vi "Create Framework Configuration.vi"(11 "Plugins":T5(array[cluster])=[{"plugin components"=[], "group configs"=[], "plugin timing"={"priority"=0, "decimation"=1, "offset"=0}, "settings"=[], "thread count"=1}]) -> (3 "Framework Configuration":T6)   [LabVIEW 2017]
uses:
  Builds/Data Sharing Framework/Current/Data Sharing Framework Core/DSF Core.lvlibp/DSF Configuration API/Public/Controls/DSF Engine Framework Configuration.ctl
  Builds/Data Sharing Framework/Current/Data Sharing Framework Core/DSF Core.lvlibp/DSF Configuration API/Public/Controls/DSF Engine Plugin Configuration.ctl
  Builds/Data Sharing Framework/Current/Data Sharing Framework Core/DSF Core.lvlibp/DSF Configuration API/Public/Controls/DSF Timing Info.ctl
  Builds/Data Sharing Framework/Current/Data Sharing Framework Core/DSF Core.lvlibp/DSF Configuration API/Public/Controls/DSF Engine Transfer Group Configuration.ctl
  Builds/Data Sharing Framework/Current/Data Sharing Framework Core/DSF Core.lvlibp/DSF Configuration API/Public/Controls/DSF Direction.ctl
  Builds/Data Sharing Framework/Current/Data Sharing Framework Core/DSF Core.lvlibp/DSF Configuration API/Public/Controls/DSF Engine Transfer Configuration.ctl
  Builds/Data Sharing Framework/Current/Data Sharing Framework Core/DSF Core.lvlibp/DSF Configuration API/Public/Controls/DSF Byte Order.ctl
  Builds/Data Sharing Framework/Current/Data Sharing Framework Core/DSF Core.lvlibp/DSF Configuration API/Public/Controls/DSF Engine Channel Configuration.ctl
  Builds/Data Sharing Framework/Current/Data Sharing Framework Core/DSF Core.lvlibp/DSF Configuration API/Public/Controls/DSF Data Type.ctl
  Builds/Data Sharing Framework/Current/Data Sharing Framework Core/DSF Core.lvlibp/DSF Configuration API/Public/Controls/DSF Settings Info.ctl
  Builds/Data Sharing Framework/Current/Data Sharing Framework Core/DSF Core.lvlibp
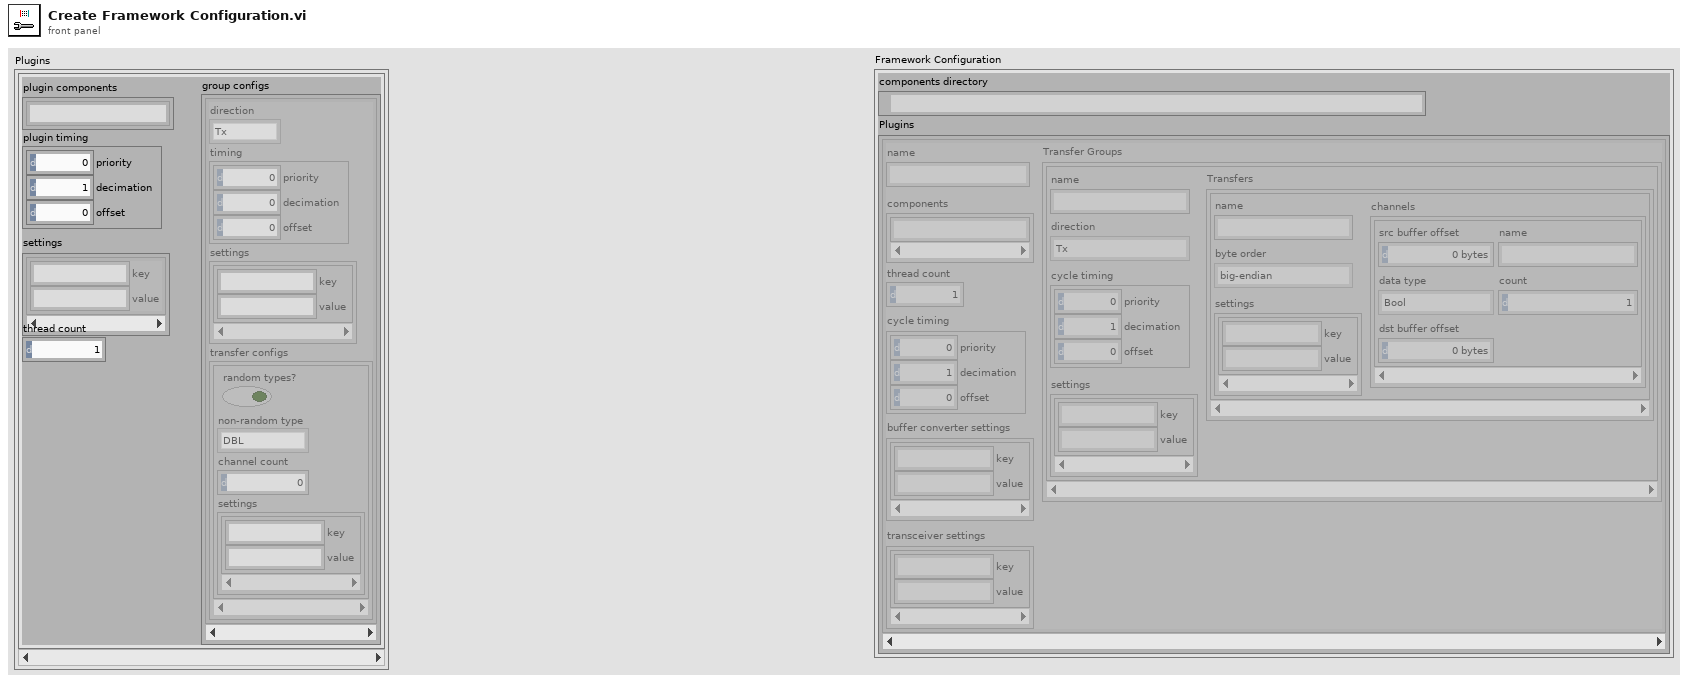
[diagram p1: front panel]
types:
  T1 = typedef "DSF Core.lvlibp/DSF Direction.ctl" = enum8{"Tx", "Rx"}
  T2 = typedef "DSF Core.lvlibp/DSF Timing Info.ctl" = cluster{"priority":u64, "decimation":u64, "offset":u64}
  T3 = typedef "DSF Core.lvlibp/DSF Settings Info.ctl" = cluster{"key":string, "value":string}[]
  T4 = typedef "DSF Core.lvlibp/DSF Data Type.ctl" = enum8{"Bool", "SGL", "DBL", "I8", "I16", "I32", "I64", "U8", "U16", "U32", "U64"}
  T5 = cluster{"plugin components":string[], "group configs":cluster{"direction":T1, "timing":T2, "settings":T3, "transfer configs":cluster{"random types?":bool, "non-random type":T4, "channel count":i32, "settings":T3}[]}[], "plugin timing":T2, "settings":T3, "thread count":i32}[]
  T6 = typedef "DSF Core.lvlibp/DSF Engine Framework Configuration.ctl" = cluster{"components directory":path, "Plugins":T7[]}
  T7 = typedef "DSF Core.lvlibp/DSF Engine Plugin Configuration.ctl" = cluster{"name":string, "components":string[], "cycle timing":T2, "Transfer Groups":T8[], "thread count":i32, "buffer converter settings":T3, "transceiver settings":T3}
  T8 = typedef "DSF Core.lvlibp/DSF Engine Transfer Group Configuration.ctl" = cluster{"name":string, "direction":T1, "cycle timing":T2, "Transfers":T9[], "settings":T3}
  T9 = typedef "DSF Core.lvlibp/DSF Engine Transfer Configuration.ctl" = cluster{"name":string, "byte order":T10, "channels":T11[], "settings":T3}
  T10 = typedef "DSF Core.lvlibp/DSF Byte Order.ctl" = enum8{"big-endian", "little-endian"}
  T11 = typedef "DSF Core.lvlibp/DSF Engine Channel Configuration.ctl" = cluster{"src buffer offset":u64, "name":string, "data type":T4, "count":u64, "dst buffer offset":u64}
  T12 = cluster{"direction":T1, "timing":T2, "settings":T3, "transfer configs":cluster{"random types?":bool, "non-random type":T4, "channel count":i32, "settings":T3}[]}[]
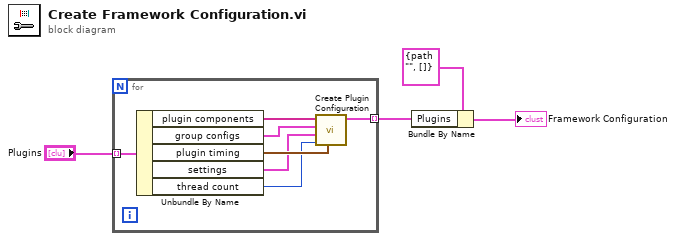
[diagram p0: block diagram]
diagram:
  n1 = for {
    tunnel: [w11] -> w1 mode=indexing
    tunnel: "Plugins" -> [w10] mode=indexing
    n2 = Unbundle By Name(w10) -> ("plugin components"=w9:string[], "group configs"=w7:T12, "plugin timing"=w8:T2, "settings"=w6:T3, "thread count"=w5:i32)
    n3 = call "Create Plugin Configuration.vi"("plugin timing"=w8, "thread count"=w5, "settings"=w6, "group configs"=w7, "plugin components"=w9) -> ("Plugin Configuration"=w11:T7)  [unwired: 6 in]
  }
  n4 = Bundle By Name(cluster=T6 {"components directory"=path "", "Plugins"=[]} ("Framework Configuration"), "Plugins"=w1) -> (→"Framework Configuration":T6)
